vi "FestoCPX.DI.Data.States.Get.vi"(8 "error in (no error)":errorcluster, 10 "CPX.DI":T1[](array[typedef])) -> (0 "error out":errorcluster, 1 "State AND":bool[](array[boolean]), 2 "State OR":bool[](array[boolean]), 3 "State":bool[](array[boolean]), 5 "FrameCounter":i32)   [LabVIEW 2016]
uses:
  FestoCPX.DI.Signal.ctl
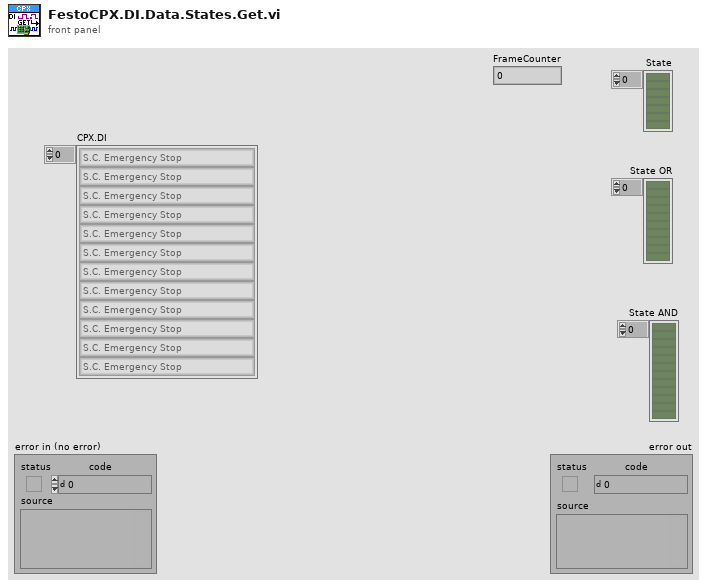
[diagram p1: front panel]
types:
  T1 = typedef "FestoCPX.DI.Signal.ctl" = enum16{"S.C. Emergency Stop", "S.C. Side Door Close", "S.C. Front Door Close", "S.C. Front Door Secured", "Button Start", "Button Stop", "Button Control", "Product Move Home", "Product Move Work", "Table Position", "Table Lock", "Product Lift A Home", "Product Lift B Home", "Product Arm OK", "Product Arm NOK", "Product Arm Work", "Revolver ID 1", "Revolver ID 2", "Revolver ID 3", "Revolver ID 4", "Revolver ID 5", "Air Pressure Inside", "Air Pressure Inlet", "Product Slot 1 A Present", "Product Slot 1 B Present", "Product Slot 2 A Present", "Product Slot 2 B Present", "Product Slot 3 A Present", "Product Slot 3 B Present", "Product Slot 4 A Present", "Product Slot 4 B Present", "Product Final A Present", "Product Final B Present", "Product Output A Present", "Product Output B Present", "Product Container OK Present", "Product Container NOK Present", "Fork ID 1", "Fork ID 2"}
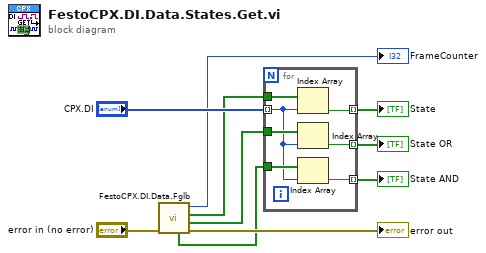
[diagram p0: block diagram]
diagram:
  n1 = call "FestoCPX.DI.Data.Fglb.vi"("error in (no error)"="error in (no error)") -> ("error out"=→"error out":errorcluster, "data OR"=w5:bool[], "data out"=w6:bool[], "FrameCounter"=→"FrameCounter":i32, "data AND"=w2:bool[])  [unwired: 6 in]
  n2 = for {
    tunnel: w6 -> [w17]
    tunnel: "CPX.DI" -> [w11] mode=indexing
    tunnel: [w16] -> w8 mode=indexing
    tunnel: w5 -> [w15]
    tunnel: [w14] -> w4 mode=indexing
    tunnel: w2 -> [w12]
    tunnel: [w13] -> w3 mode=indexing
    n3 = Index Array(array=w17, index=w11) -> (element=w16:bool)
    n4 = Index Array(array=w15, index=w11) -> (element=w14:bool)
    n5 = Index Array(array=w12, index=w11) -> (element=w13:bool)
  }
  "State" <- w8
  "State OR" <- w4
  "State AND" <- w3
